vi "callFunction.vi"(6 "timeout (ms)":i32=-1, 7 "object":string, 8 "error in (no error)":errorcluster, 9 "argument list in":T1[](array[typedef]), 10 "function":string, 11 "LabVIEW-Python-Interface in":refnum<class "PyLVi.lvclass">) -> (0 "error out":errorcluster, 1 "return list":T1[](array[typedef]), 3 "LabVIEW-Python-Interface out":refnum<class "PyLVi.lvclass">)   [LabVIEW 2016, in "PyLVi.lvlib" / "PyLVi.lvclass"]
uses:
  PyLVi.lvclass
  Controls/ArgumentStructure.ctl
  Controls/DescriptorStructure.ctl
  Controls/FunctionStructure.ctl
panel:
  out "return message":string
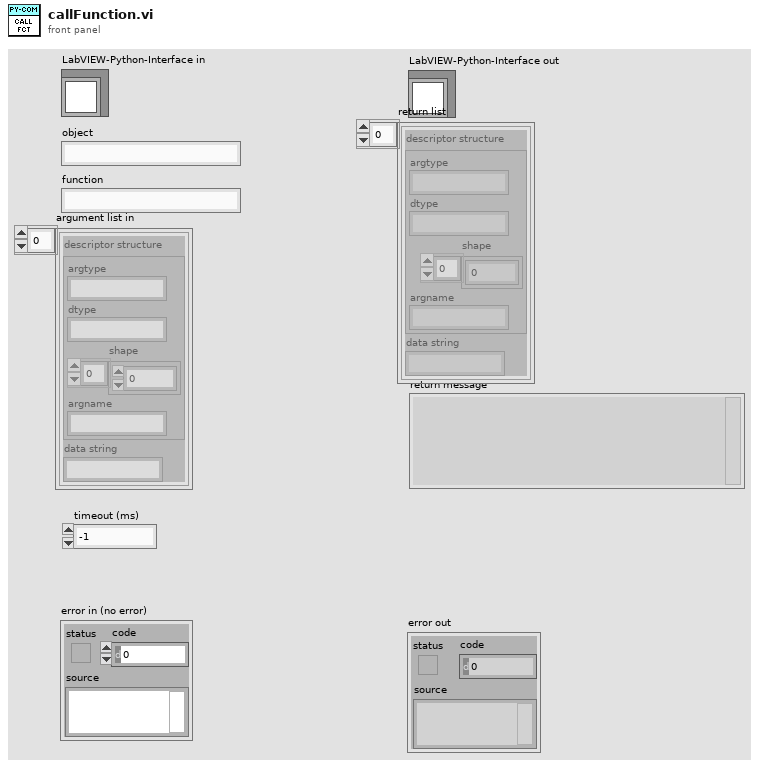
[diagram p1: front panel]
types:
  T1 = typedef "PyLVi.lvlib/PyLVi.lvclass/ArgumentStructure.ctl" = cluster{"descriptor structure":T2, "data string":string}
  T2 = typedef "PyLVi.lvlib/PyLVi.lvclass/DescriptorStructure.ctl" = cluster{"argtype":string, "dtype":string, "shape":u32[], "argname":string}
  T3 = typedef "PyLVi.lvlib/PyLVi.lvclass/FunctionStructure.ctl" = cluster{"obj":string, "fct":string}
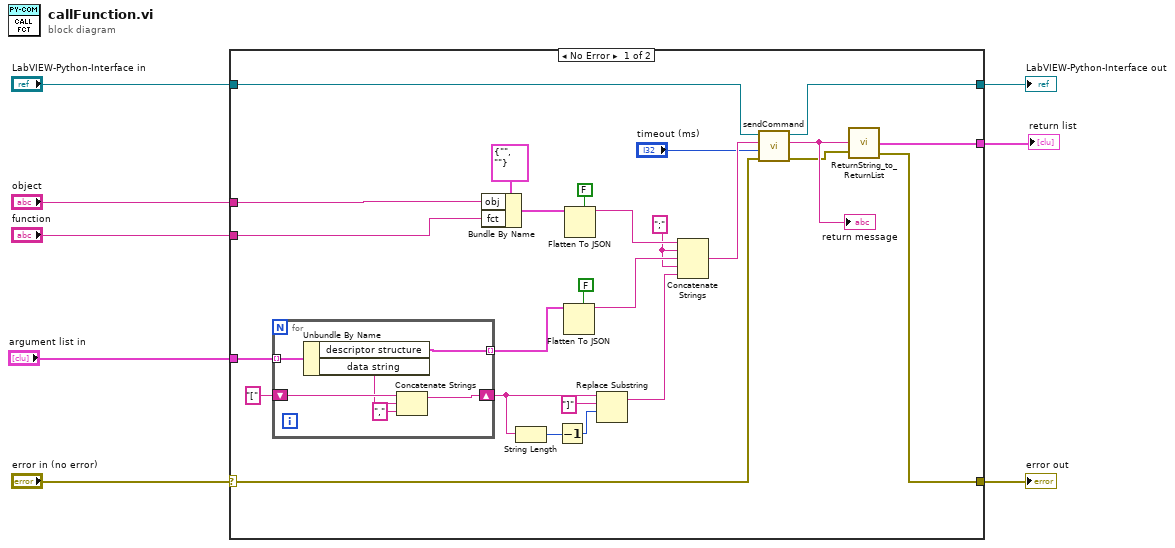
[diagram p0: block diagram]
diagram:
  n1 = case shown="No Error" "error in (no error)" {
    selector: "error in (no error)" -> [w11 w41]
    tunnel: [w10 w41] -> w7
    tunnel: [w33 w42] -> w5
    tunnel: "LabVIEW-Python-Interface in" -> [w34 w42]
    tunnel: "object" -> [w31 _]
    tunnel: "function" -> [w30 _]
    tunnel: "argument list in" -> [w22 _]
    tunnel: [w19 _] -> w1
    frame No Error {
      w24 = ";" ("string")
      n2 = for {
        tunnel: w22 -> [w40] mode=indexing
        tunnel: [w39] -> w21 mode=indexing
        shift-right: [w38] -> w16
        shift-left: "[" ("string") -> [w37]
        n3 = Unbundle By Name(w40) -> ("descriptor structure"=w39:T2, "data string"=w36:string)
        n4 = Concatenate Strings(w37, w36, "," ("string")) -> (w38:string)
      }
      n5 = Bundle By Name(cluster=T3 {"obj"="", "fct"=""} ("function structure"), "obj"=w31, "fct"=w30) -> (w29:T3)
      n6 = String Length(string=w16) -> (length=w15:i32)
      n7 = Decrement(x=w15) -> (x-1=w14:i32)
      n8 = Flatten To JSON(enable LabVIEW extensions? (T)=FALSE, anything=w21) -> (JSON string=w25:string)  [unwired: 1 in, 1 out]
      n9 = Flatten To JSON(enable LabVIEW extensions? (T)=FALSE, anything=w29) -> (JSON string=w27:string)  [unwired: 1 in, 1 out]
      n10 = Replace Substring(3:w14, 4:"]" ("string"), 5:w16) -> (1:w13:string)  [unwired: 1 in, 1 out]
      n11 = Concatenate Strings(w27, w24, w25, w24, w13) -> (w23:string)
      n12 = call "sendCommand.vi"("error in (no error)"=w11, "timeout (ms)"="timeout (ms)", "command"=w23, "LabVIEW-Python-Interface in"=w34) -> ("error out"=w12:errorcluster, "data"=w20:string, "LabVIEW-Python-Interface out"=w33:refnum<class "PyLVi.lvclass">)  [unwired: 4 in, 1 out]
      "return message" <- w20
      n13 = call "ReturnString_to_ReturnList.vi"("error in (no error)"=w12, "return string"=w20) -> ("error out"=w10:errorcluster, "return list"=w19:T1[])  [unwired: 2 in]
    }
    frame Error {
    }
  }
  "error out" <- w7
  "LabVIEW-Python-Interface out" <- w5
  "return list" <- w1
